vi "Write listening net address.vi"(8 "error in (no error)":errorcluster, 10 "listening net address":u32, 11 "TCP Slave in":refnum<class "TCP Slave.lvclass">) -> (0 "error out":errorcluster, 3 "TCP Slave out":refnum<class "TCP Slave.lvclass">)   [LabVIEW 2021, in "TCP Slave.lvclass"]
uses:
  TCP Slave.lvclass
  TCP Slave.lvclass/TCP Slave.ctl
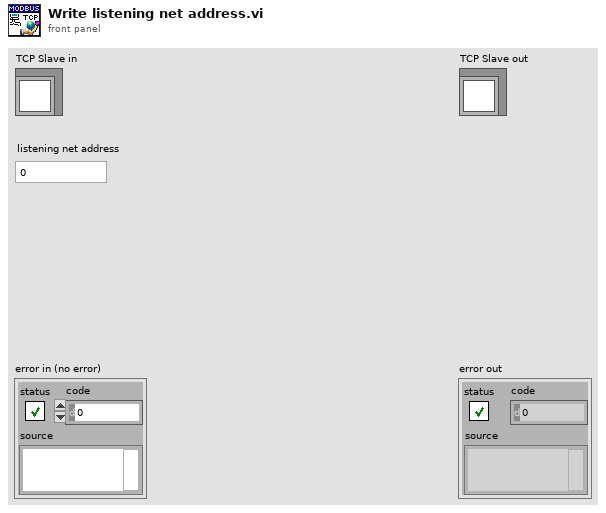
[diagram p1: front panel]
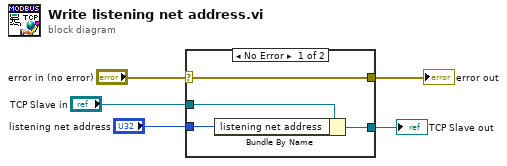
[diagram p0: block diagram]
diagram:
  n1 = case shown="No Error" "error in (no error)" {
    selector: "error in (no error)" -> [w9 w10]
    tunnel: [w9 w10] -> w4
    tunnel: [w7 w11] -> w2
    tunnel: "TCP Slave in" -> [w8 w11]
    tunnel: "listening net address" -> [w6 _]
    frame No Error {
      n2 = Bundle By Name(cluster=w8, "listening net address"=w6) -> (w7:refnum<class "TCP Slave.lvclass">)
    }
    frame Error {
    }
  }
  "error out" <- w4
  "TCP Slave out" <- w2
